vi "Voice coil and camera trigger.vi"() -> ()   [LabVIEW 2020]
uses:
  <vilib>/DAQmx/write.llb/DAQmx Write (Analog Wfm 1Chan NSamp).vi
  <vilib>/DAQmx/create/channels.llb/DAQmx Create Channel (AO-Voltage-Basic).vi
  <vilib>/DAQmx/configure/timing.llb/DAQmx Timing (Use Waveform).vi
  <vilib>/DAQmx/miscellaneous.llb/DAQmx Fill In Error Info.vi
  <vilib>/measure/NI_MABase.lvlib
panel:
  in  "Stop 2":bool
  out "LabVIEW generated Sawtooth input (blue) and Camera trigger (red)":waveform(dbl)(graph)={"t0"=timestamp(0 s since 1904-01-01), "dt"=0.001, "Y"=array[1000 elements]}
  in  "Sawtooth Offset (mv)":dbl format="%.2p"
  in  "Exposure time (ms)":dbl=1000.0
  out "# Samples written per channel":u32=1000
  in  "Sawtooth Phase":dbl=180.0 format="%.2p"
  in  "Sawtooth Amplitude (mv)":dbl format="%.2p"
  # "Sawtooth signal has to be smooth around the edges"
  # "Fs= sampling rate in samples per second\n#s= number of samples in the waveform"
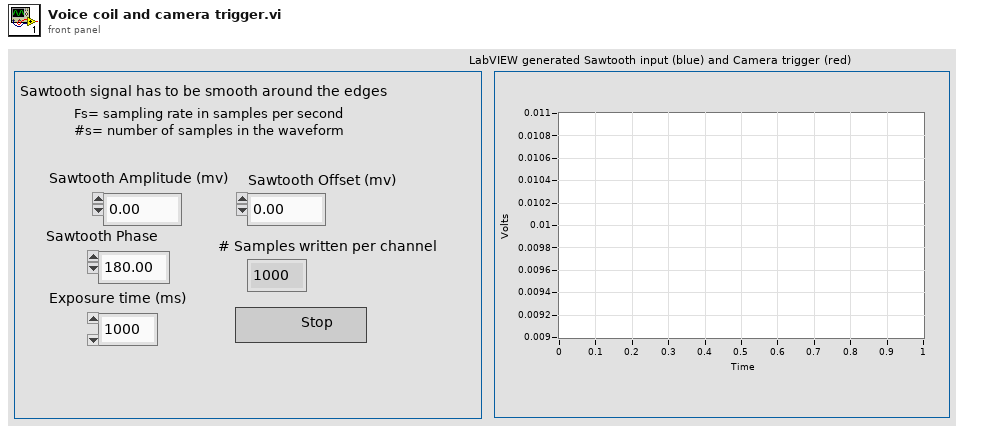
[diagram p1: front panel]
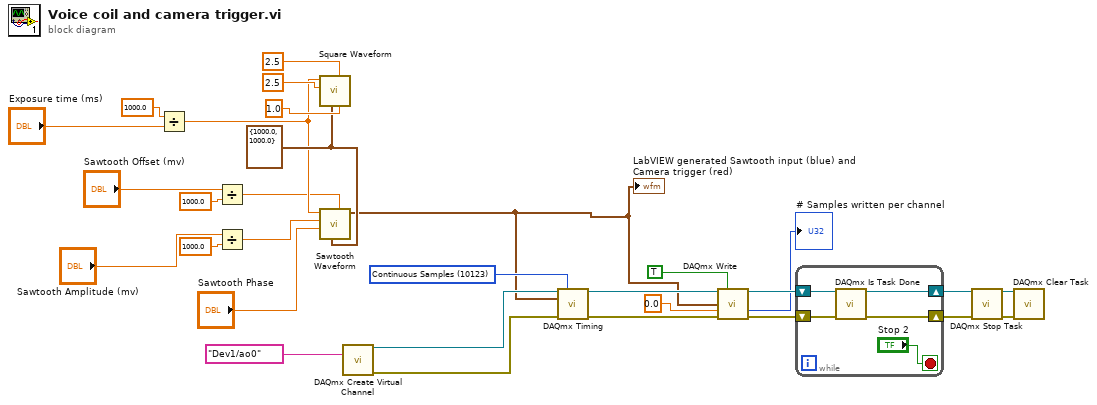
[diagram p0: block diagram]
diagram:
  w10 = cluster{"Fs":dbl, "#s":dbl} {"Fs"=1000.0, "#s"=1000.0} ("sampling info")
  w25 = 10123 items=["Finite Samples"=10178, "Continuous Samples"=10123, "Hardware Timed Single Point"=12522] ("sample mode")
  n1 = Divide(x=1000.0, y="Exposure time (ms)") -> (x/y=w8:dbl)
  n2 = Divide(x="Sawtooth Offset (mv)", y=1000.0) -> (x/y=w7:dbl)
  n3 = Divide(x="Sawtooth Amplitude (mv)", y=1000.0) -> (x/y=w2:dbl)
  n4 = call <vilib>:"Square Waveform.vi"("duty cycle (%)"=1.0, "offset"=2.5, "sampling info"=w10, "amplitude"=2.5, "frequency"=w8) -> ()  [unwired: 5 in, 2 out]
  n5 = call <vilib>:"Sawtooth Waveform.vi"("offset"=w7, "sampling info"=w10, "phase"="Sawtooth Phase", "amplitude"=w2, "frequency"=w8) -> ("signal out"=w1:waveform(dbl))  [unwired: 5 in, 1 out]
  "LabVIEW generated Sawtooth input (blue) and Camera trigger (red)" <- w1
  n6 = call-poly <vilib>:"DAQmx Create Virtual Channel.vi"("physical channels"=tag "Dev1/ao0") -> ("task out"=w27:refnum<k21>, "error out"=w26:errorcluster)  [unwired: 13 in]
  n7 = call-poly <vilib>:"DAQmx Timing.vi"("task/channels in"=w27, "sample mode"=w25, "waveform"=w1, "error in"=w26) -> ("task out"=w22:refnum<k21>, "error out"=w21:errorcluster)  [unwired: 10 in]
  n8 = call-poly <vilib>:"DAQmx Write.vi"("task/channels in"=w22, "auto start"=TRUE, "data"=w1, "timeout"=0.0, "error in"=w21) -> ("task out"=w23:refnum<k21>, "number of samples written per channel"=→"# Samples written per channel":u32, "error out"=w24:errorcluster)  [unwired: 8 in]
  n9 = while {
    shift-right: [w32] -> w18
    shift-left: w23 -> [w35]
    shift-right: [w33] -> w19
    shift-left: w24 -> [w34]
    stop <- "Stop 2" stop-if-true
    n10 = call <vilib>:"DAQmx Is Task Done.vi"("task/channels in"=w35, "error in"=w34) -> ("task out"=w32:refnum<k21>, "error out"=w33:errorcluster)  [unwired: 11 in, 1 out]
  }
  n11 = call <vilib>:"DAQmx Stop Task.vi"("task/channels in"=w18, "error in"=w19) -> ("task out"=w28:refnum<k21>, "error out"=w29:errorcluster)  [unwired: 12 in]
  n12 = call <vilib>:"DAQmx Clear Task.vi"("task in"=w28, "error in"=w29) -> ()  [unwired: 13 in, 1 out]
